vi "init.vi"(8 "error in (no error)":errorcluster, 11 "FlowControlValveCompensator_Lateral in":refnum<class "FlowControlValveCompensator_Lateral.lvclass">) -> (0 "error out":errorcluster, 3 "FlowControlValveCompensator_Lateral out":refnum<class "FlowControlValveCompensator_Lateral.lvclass">)   [LabVIEW 2013, in "FlowControlValveCompensator_Lateral.lvclass"]
uses:
  FlowControlValveCompensator_Lateral.lvclass
  Configuration/FlowControlValveCompensator.ctl
  Configuration/PIDGains.ctl
  Configuration/FlowControlValveOutputRange.ctl
  FlowControlValveCompensator/FlowControlValveCompensator.lvclass/FlowControlValveCompensator.ctl
  ConfigurationThisComponent/ConfigurationThisComponent.lvclass
  FlowControlValveCompensator/FlowControlValveCompensator.lvclass
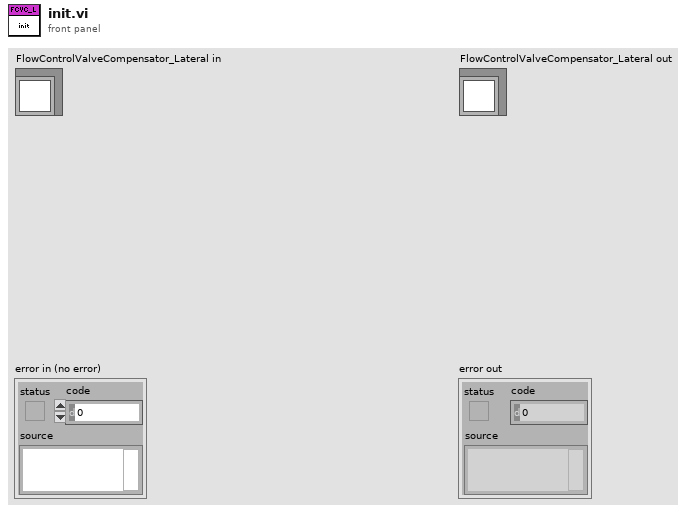
[diagram p1: front panel]
types:
  T1 = typedef "FlowControlValveCompensator.ctl" = cluster{"PID Gains":T2, "Flow Control Valve Output Range":T3}
  T2 = typedef "PIDGains.ctl" = cluster{"Proportional Gain (Kc)":dbl, "Integral Time (Ti, min)":dbl, "Derivative Time (Td, min)":dbl}
  T3 = typedef "FlowControlValveOutputRange.ctl" = cluster{"High":dbl[unit], "Low":dbl[unit]}
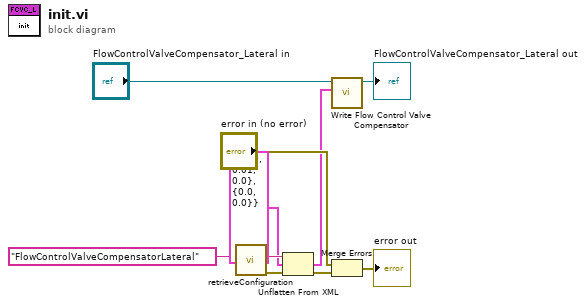
[diagram p0: block diagram]
diagram:
  n1 = call "retrieveConfiguration.vi"("configName"="FlowControlValveCompensatorLateral") -> ("error out"=w8:errorcluster, "xmlConfig"=w7:string)  [unwired: 8 in, 1 out]
  n2 = Unflatten From XML(xml string=w7, type=T1 {"PID Gains"={"Proportional Gain (Kc)"=1.0, "Integral Time (Ti, min)"=0.01, "Derivative Time (Td, min)"=0.0}, "Flow Control Valve Output Range"={"High"=0.0, "Low"=0.0}} ("Flow Control Valve Compensator"), error in (no error)=w8) -> (value=w1:T1, error out=w10:errorcluster)
  n3 = call "Write Flow Control Valve Compensator.vi"("Flow Control Valve Compensator"=w1, "FlowControlValveCompensator in"="FlowControlValveCompensator_Lateral in") -> ("FlowControlValveCompensator out"=→"FlowControlValveCompensator_Lateral out":refnum<class "FlowControlValveCompensator_Lateral.lvclass">)  [unwired: 9 in]
  n4 = Merge Errors("error in (no error)", w10) -> (→"error out":errorcluster)
